vi "Event Polarity Discriminator.vi"(5 "Integrations vs. Time":waveform(dbl)[](array[waveform]), 7 "Integration Level (V ms)":dbl, 9 "Time Difference Threshold (ms)":dbl=0.0001) -> (3 "Time Differences":dbl[](array[numeric]), 8 "Event Polarity":u32, 14 "Average Time Diference":dbl)   [LabVIEW 2013, in "Breakdown Acoustics Controls.lvlib"]
uses:
  <vilib>/express/express signal manip/TriggerBlock.llb/triggerSense.ctl
  Breakdown Acoustics Controls.lvlib
panel:
  out "Satisfied":bool
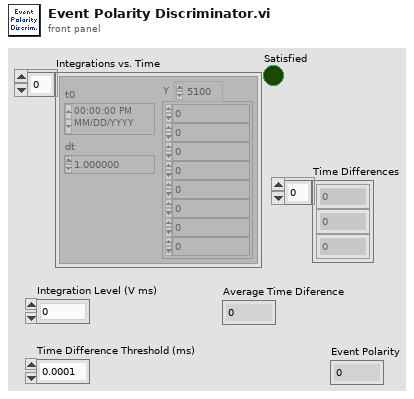
[diagram p1: front panel]
types:
  T1 = typedef "triggerSense.ctl" = enum32{"Rising", "Rising or Falling", "Falling"}
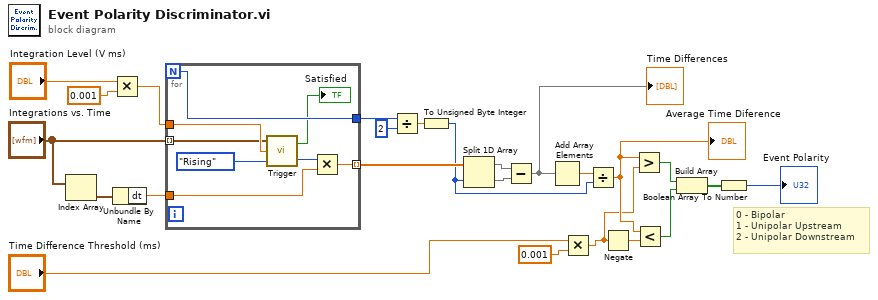
[diagram p0: block diagram]
diagram:
  # "0 - Bipolar\n1 - Unipolar Upstream \n2 - Unipolar Downstream"
  n1 = Index Array(array="Integrations vs. Time") -> (element=w8:waveform(dbl))  [unwired: 1 in]
  n2 = Multiply(x="Integration Level (V ms)", y=0.001) -> (x*y=w5:dbl)
  n3 = Unbundle By Name(w8) -> ("dt"=w7:dbl)
  n4 = for {
    N -> [w26]
    tunnel: w5 -> [w31]
    tunnel: [w27] -> w24 mode=indexing
    tunnel: "Integrations vs. Time" -> [w30] mode=indexing
    tunnel: [w26] -> w23
    tunnel: w7 -> [w28]
    n5 = call "Trigger.vi"("Sense"=triggerSense."Rising", "Threshold"=w31, "Waveform"=w30) -> ("Index"=w29:u32, "Satisfied"=→"Satisfied":bool)  [unwired: 1 in]
    n6 = Multiply(x=w29, y=w28) -> (x*y=w27:dbl)
  }
  n7 = Divide(x=w23, y=2) -> (x/y=w21:dbl)
  n8 = To Unsigned Byte Integer(number=w21) -> (unsigned 8bit integer=w11:u8)
  n9 = Split 1D Array(array=w24, index=w11) -> (first subarray=w20:dbl[], second subarray=w19:dbl[])
  n10 = Subtract(x=w20, y=w19) -> (x-y=w13:dbl[])
  "Time Differences" <- w13
  n11 = Add Array Elements(numeric array=w13) -> (sum=w18:dbl)
  n12 = Multiply(x="Time Difference Threshold (ms)", y=0.001) -> (x*y=w1:dbl)
  n13 = Divide(x=w18, y=w11) -> (x/y=w17:dbl)
  "Average Time Diference" <- w17
  n14 = Negate(x=w1) -> (-x=w16:dbl)
  n15 = Greater?(x=w17, y=w1) -> (0:w15:bool)
  n16 = Less?(x=w17, y=w16) -> (x < y?=w14:bool)
  n17 = Build Array(w15, w14) -> (w12:bool[])
  n18 = Boolean Array To Number(Boolean array=w12) -> (number=→"Event Polarity":u32)
